vi "Set Stream ID.vi"(8 "error in (no error)":errorcluster, 10 "stream id":u16, 11 "Transfer Configuration in":refnum<class "Transfer Configuration.lvclass">) -> (0 "error out":errorcluster, 3 "Transfer Configuration out":refnum<class "Transfer Configuration.lvclass">)   [LabVIEW 2017, in "PXImc.lvlib" / "Transfer Configuration.lvclass"]
uses:
  Transfer Configuration.lvclass
  Transfer Configuration.lvclass/Transfer Configuration.ctl
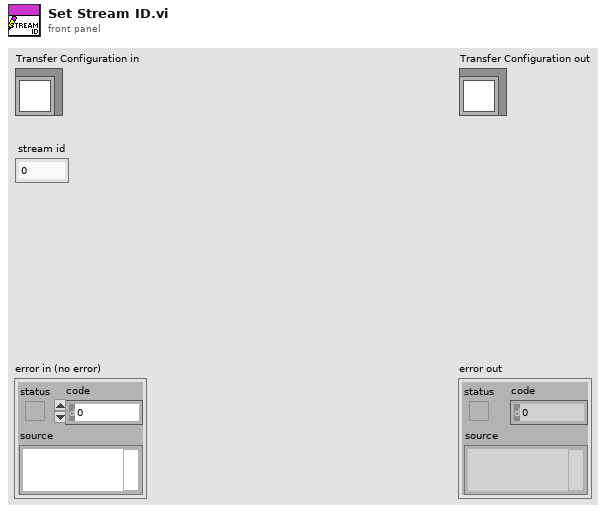
[diagram p1: front panel]
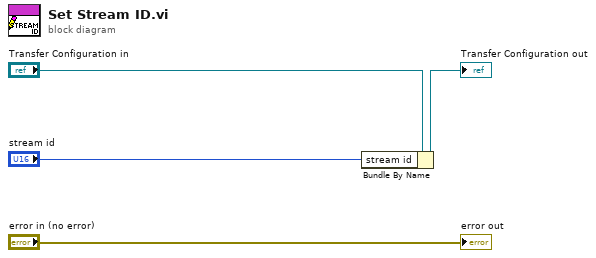
[diagram p0: block diagram]
diagram:
  n1 = Bundle By Name(cluster="Transfer Configuration in", "stream id"="stream id") -> (→"Transfer Configuration out":refnum<class "Transfer Configuration.lvclass">)
  "error out" <- "error in (no error)"
